vi "quiz 3.vi"() -> ()   [LabVIEW 2017]
panel:
  out "text":string
  in  "Tab Control":enum32{"Page 1", "Page 2"}(tab)
  in  "Ingresar":bool
  in  "usuario":string
  in  "Contraseña":string
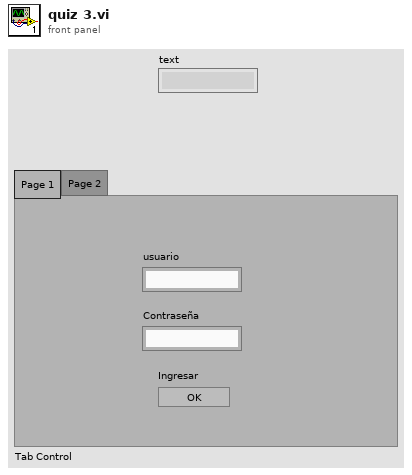
[diagram p1: front panel]
types:
  T1 = enum16{"open", "replace", "create", "open or create", "replace or create", "replace or create with confirmation"}
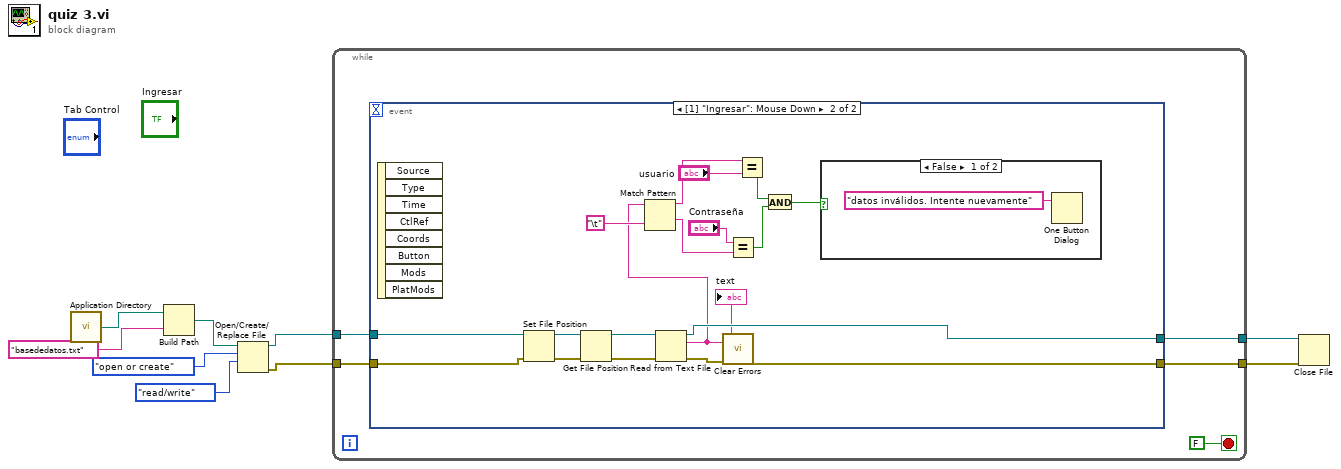
[diagram p0: block diagram]
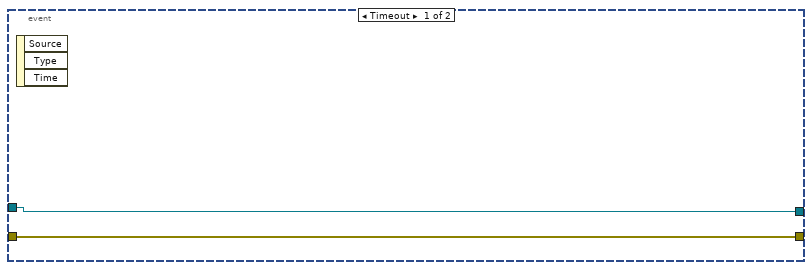
[diagram p2: hidden frame]
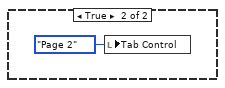
[diagram p3: hidden frame]
diagram:
  n1 = call <vilib>:"Application Directory.vi"() -> ("Application Directory"=w2:path)
  n2 = Build Path(base path=w2, name or relative path="basededatos.txt") -> (appended path=w3:path)
  n3 = Open/Create/Replace File(file path (use dialog)=w3, operation (0:open)=T1."open or create", access (0:read/write)=enum16{"read/write", "read-only", "write-only"}."read/write") -> (refnum out=w9:refnum<file>, error out=w8:errorcluster)  [unwired: 3 in, 1 out]
  n4 = while {
    tunnel: w9 -> [w14]
    tunnel: w8 -> [w13]
    tunnel: [w12] -> w5
    tunnel: [w11] -> w4
    stop <- FALSE stop-if-true
    n5 = event shown="[1] \"Ingresar\": Mouse Down" {
      selector: _ -> [_ _]
      dyn-events: _ -> [_ _]
      timeout: _ -> [_ _]
      tunnel: w14 -> [w15 w29]
      tunnel: w13 -> [w16 w28]
      tunnel: [w16 w27] -> w12
      tunnel: [w15 w26] -> w11
      event Timeout {
        n6 = event-data() -> ()  [unwired: 1 in, 3 out]
      }
      event "Ingresar": Mouse Down {
        n7 = event-data() -> ()  [unwired: 1 in, 8 out]
        n8 = Set File Position(refnum=w29, error in=w28) -> (refnum out=w34:refnum<file>, error out=w32:errorcluster)  [unwired: 2 in]
        n9 = Get File Position(4:w32, 7:w34) -> (0:w31:errorcluster, 3:w33:refnum<file>)  [unwired: 1 out]
        n10 = Read from Text File(file (use dialog)=w33, error in=w31) -> (refnum out=w26:refnum<file>, text=w24:string, error out=w30:errorcluster)  [unwired: 2 in, 1 out]
        "text" <- w24
        n11 = Match Pattern(string=w24, regular expression="\t") -> (before substring=w23:string, after substring=w22:string)  [unwired: 1 in, 2 out]
        n12 = call <vilib>:"Clear Errors.vi"("error in (no error)"=w30) -> ("error out"=w27:errorcluster)  [unwired: 5 in, 1 out]
        n13 = Equal?(x="Contraseña", y=w22) -> (x = y?=w18:bool)
        n14 = Equal?(x=w23, y="usuario") -> (x = y?=w19:bool)
        n15 = And(x=w19, y=w18) -> (x .and. y?=w17:bool)
        n16 = case shown="False" w17 {
          frame False {
            n17 = One Button Dialog(message="datos inválidos. Intente nuevamente") -> ()  [unwired: 1 in, 1 out]
          }
          frame True {
            n18 = local write "Tab Control"(enum32{"Page 1", "Page 2"}."Page 2" ("Tab Control")) -> ()
          }
        }
      }
    }
  }
  n19 = Close File(refnum=w4, error in=w5) -> ()  [unwired: 2 out]
